vi "Controller LNLS Control BPM Communication Loop.vi"(7 "Sync Objects":T1, 8 "error in (no error)":errorcluster, 11 "FOFB Configuration":T4={"FOFB Parameters"={"Network"={"FOFB Controller IP"="", "LNLS Control Network IP"="", "LNLS Control Network Power Supplies TCP Port"=0, "LNLS Control Network FOFB Configuration TCP Port"=0, "LNLS Control Network BPMs TCP Port"=0, "Data Server TCP Port"=0, "Monitoring Data TCP Port"=0, "Configuration GUI TCP Port"=0, "Storage Data TCP Port"=0, "Fast Command TCP Port"=0, "TCP Listening Timeout"=0, "Request Setpoints Rate"=0}, "Fast Acquisition"={"Acquisition Period"=0, "Data Buffer Size"=0, "Monitoring Period"=0}, "Response Matrix Measurement"={"Step Amplitude"=0.0, "Time Between Steps"=0, "Step Duration"=0, "Number of Averages"=0}, "Correction Algorithm"={"Correction Period"=0, "Reference Orbit Path"=path "", "Response Matrix Path"=path "", "Correction Matrix Path"=path "", "PID Horizontal Gain"=0.0, "PID Vertical Gain"=0.0, "PID Horizontal Integral Time"=0.0, "PID Vertical Integral Time"=0.0, "PID Horizontal Derivative Time"=0.0, "PID Vertical Derivative Time"=0.0, "Beam Current FOFB Threshold"=0.0, "Decouple H-V"=FALSE, "Use Additional BPM LPF"=FALSE, "BPM LPF Cutoff"=0.0}, "Acquisition Network"=[], "Actuation Network"=[]}, "Number of Acquisition Chassis"=0, "Number of Actuation Chassis"=0, "Number of BPM Readings"=0, "BPM Reading Names"=[], "Selected BPM Readings"=[0, 1, 2, 3, 4, 5, 6, 7, 8, 9, 10, 11, 12, 13, 14, 15, 16, 17, 18, 19, 20, 21, 22, 23, 24, 25, 26, 27, 28, 29, 30, 31, 32, 33, 34, 35, 36, 37, 38, 39, 40, 41, 42, 43, 44, 45, 46, 47, 48, 49], "Number of Correctors"=0, "Corrector Names"=[], "Selected Correctors"=[0, 1, 2, 3, 4, 5, 6, 7, 8, 9, 10, 11, 12, 13, 14, 15, 16, 17, 18, 19, 20, 21, 22, 23, 24, 25, 26, 27, 28, 29, 30, 31, 32, 33, 34, 35, 36, 37, 38, 39, 40, 41, 42, 43, 44, 45, 46, 47, 48, 49], "Reference Orbit"=[], "Response Matrix"=[], "Correction Matrix"=[], "Acquisition Chassis Names"=[], "Actuation Chassis Names"=[], "Acquisition Variables"=[], "Actuation Variables"=[], "PS Matrix Mapping"=[], "Inverse PS Matrix Mapping"=[], "BPM Matrix Mapping"=[], "Inverse BPM Matrix Mapping"=[], "Response Matrix Beam Energy (MeV)"=0.0, "PID Parameters"=[], "BPM Planes"=[], "Corrector Planes"=[], "RMM Step Factor"=[]}) -> (0 "error out":errorcluster)   [LabVIEW 2011, in "Controller Global Variables.lvlib"]
uses:
  Controller Global Variables.lvlib
  Types Definitions/Type FOFB Configuration.ctl
  Types Definitions/Type FOFB Parameters.ctl
  Types Definitions/Type Network Configuration.ctl
  Types Definitions/Type FA Configuration.ctl
  Types Definitions/Type Response Matrix Measurement Configuration.ctl
  Types Definitions/Type Correction Algorithm Configuration.ctl
  Types Definitions/Type Acquisition Network Configuration.ctl
  Types Definitions/Type Actuation Network Configuration.ctl
  Types Definitions/Type PID Parameters.ctl
  Types Definitions/Type Synchronization Objects.ctl
  Types Definitions/Type Blocking Synchronization Objects.ctl
  Types Definitions/Type Monitoring Data.ctl
  Types Definitions/Type Operation Mode State.ctl
  Types Definitions/Type Diagnostics Data.ctl
  Types Definitions/Type CPU Loads Array.ctl
  Types Definitions/Type CPU Loads.ctl
  Types Definitions/Type Non-blocking Synchronization Objects.ctl
  Types Definitions/Type FOFB Variables.ctl
  Types Definitions/Type Actuation State.ctl
  Types Definitions/Type TCP State.ctl
  <vilib>/Platform/TimedLoop/XDataNode/timing_clust.ctl
  <vilib>/Platform/TimedLoop/XDataNode/nitl_modes.ctl
  <vilib>/Platform/TimedLoop/XDataNode/wakeup.ctl
  Controller Global Variables/Monitoring Data.vi
  <vilib>/Platform/TimedLoop/XDataNode/XDataNode.xnode
  Type Definitions.lvlib
  LNLS Control VIs.lvlib
  Misc VIs.lvlib
  <vilib>/Platform/TimedLoop/XDataNode/XDNodeRunTimeDep.lvlib
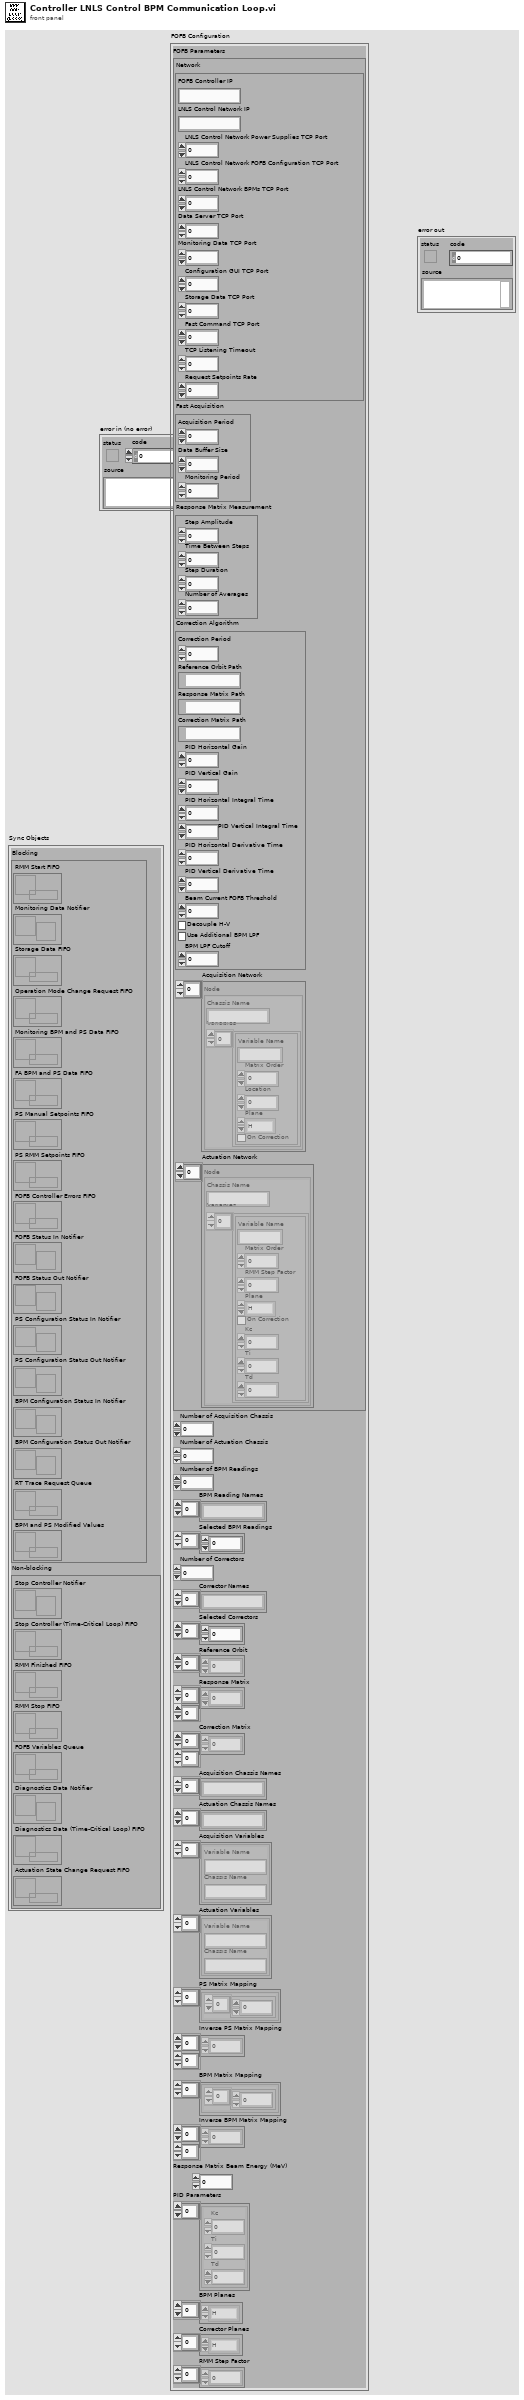
[diagram p1: front panel]
types:
  T1 = typedef "Type Definitions.lvlib/Type Synchronization Objects.ctl" = cluster{"Blocking":T2, "Non-blocking":T3}
  T2 = typedef "Type Definitions.lvlib/Type Blocking Synchronization Objects.ctl" = cluster{"RMM Start FIFO":refnum<k33>, "Monitoring Data Notifier":refnum<notifier>, "Storage Data FIFO":refnum<queue>, "Operation Mode Change Request FIFO":refnum<k33>, "Monitoring BPM and PS Data FIFO":refnum<k33>, "FA BPM and PS Data FIFO":refnum<k33>, "PS Manual Setpoints FIFO":refnum<k33>, "PS RMM Setpoints FIFO":refnum<k33>, "FOFB Controller Errors FIFO ":refnum<k33>, "FOFB Status In Notifier":refnum<notifier>, "FOFB Status Out Notifier":refnum<notifier>, "PS Configuration Status In Notifier":refnum<notifier>, "PS Configuration Status Out Notifier":refnum<notifier>, "BPM Configuration Status In Notifier":refnum<notifier>, "BPM Configuration Status Out Notifier":refnum<notifier>, "RT Trace Request Queue":refnum<queue>, "BPM and PS Modified Values":refnum<k33>}
  T3 = typedef "Type Definitions.lvlib/Type Non-blocking Synchronization Objects.ctl" = cluster{"Stop Controller Notifier":refnum<notifier>, "Stop Controller (Time-Critical Loop) FIFO":refnum<k33>, "RMM Finished FIFO":refnum<k33>, "RMM Stop FIFO":refnum<k33>, "FOFB Variables Queue":refnum<queue>, "Diagnostics Data Notifier":refnum<notifier>, "Diagnostics Data (Time-Critical Loop) FIFO":refnum<k33>, "Actuation State Change Request FIFO":refnum<k33>}
  T4 = typedef "Type Definitions.lvlib/Type FOFB Configuration.ctl" = cluster{"FOFB Parameters":T5, "Number of Acquisition Chassis":i32, "Number of Actuation Chassis":i32, "Number of BPM Readings":i32, "BPM Reading Names":string[], "Selected BPM Readings":u32[], "Number of Correctors":i32, "Corrector Names":string[], "Selected Correctors":u32[], "Reference Orbit":dbl[], "Response Matrix":dbl[][], "Correction Matrix":dbl[][], "Acquisition Chassis Names":string[], "Actuation Chassis Names":string[], "Acquisition Variables":cluster{"Variable Name":string, "Chassis Name":string}[], "Actuation Variables":cluster{"Variable Name":string, "Chassis Name":string}[], "PS Matrix Mapping":cluster{u32[]}[], "Inverse PS Matrix Mapping":u32[][], "BPM Matrix Mapping":cluster{u32[]}[], "Inverse BPM Matrix Mapping":u32[][], "Response Matrix Beam Energy (MeV)":dbl, "PID Parameters":T12[], "BPM Planes":enum8{"H", "V"}[], "Corrector Planes":enum8{"H", "V"}[], "RMM Step Factor":dbl[]}
  T5 = typedef "Type Definitions.lvlib/Type FOFB Parameters.ctl" = cluster{"Network":T6, "Fast Acquisition":T7, "Response Matrix Measurement":T8, "Correction Algorithm":T9, "Acquisition Network":T10, "Actuation Network":T11}
  T6 = typedef "Type Definitions.lvlib/Type Network Configuration.ctl" = cluster{"FOFB Controller IP":string, "LNLS Control Network IP":string, "LNLS Control Network Power Supplies TCP Port":u16, "LNLS Control Network FOFB Configuration TCP Port":u16, "LNLS Control Network BPMs TCP Port":u16, "Data Server TCP Port":u16, "Monitoring Data TCP Port":u16, "Configuration GUI TCP Port":u16, "Storage Data TCP Port":u16, "Fast Command TCP Port":u16, "TCP Listening Timeout":i32, "Request Setpoints Rate":u16}
  T7 = typedef "Type Definitions.lvlib/Type FA Configuration.ctl" = cluster{"Acquisition Period":u32, "Data Buffer Size":u32, "Monitoring Period":u32}
  T8 = typedef "Type Definitions.lvlib/Type Response Matrix Measurement Configuration.ctl" = cluster{"Step Amplitude":dbl, "Time Between Steps":u32, "Step Duration":u32, "Number of Averages":u32}
  T9 = typedef "Type Definitions.lvlib/Type Correction Algorithm Configuration.ctl" = cluster{"Correction Period":u32, "Reference Orbit Path":path, "Response Matrix Path":path, "Correction Matrix Path":path, "PID Horizontal Gain":dbl, "PID Vertical Gain":dbl, "PID Horizontal Integral Time":dbl, "PID Vertical Integral Time":dbl, "PID Horizontal Derivative Time":dbl, "PID Vertical Derivative Time":dbl, "Beam Current FOFB Threshold":dbl, "Decouple H-V":bool, "Use Additional BPM LPF":bool, "BPM LPF Cutoff":dbl}
  T10 = typedef "Type Definitions.lvlib/Type Acquisition Network Configuration.ctl" = cluster{"Chassis Name":string, "Variables":cluster{"Variable Name":string, "Matrix Order":u32, "Location":dbl, "Plane":enum8{"H", "V"}, "On Correction":bool}[]}[]
  T11 = typedef "Type Definitions.lvlib/Type Actuation Network Configuration.ctl" = cluster{"Chassis Name":string, "Variables":cluster{"Variable Name":string, "Matrix Order":u32, "RMM Step Factor":dbl, "Plane":enum8{"H", "V"}, "On Correction":bool, "Kc":dbl, "Ti":dbl, "Td":dbl}[]}[]
  T12 = typedef "Type Definitions.lvlib/Type PID Parameters.ctl" = cluster{"Kc":fxp<+/-,16,8>, "Ti":fxp<+/-,16,8>, "Td":fxp<+/-,16,8>}
  T13 = typedef "Type Definitions.lvlib/Type TCP State.ctl" = enum16{"Idle", "Wait Connection", "Read Data", "Process Data", "Write Data", "Close Connection"}
  T14 = typedef "XDNodeRunTimeDep.lvlib/timing_clust.ctl" = cluster{"Expected End [f-1]":u64, "Actual End [f-1]":u64, "Finished Late? [f-1]":bool, "Expected End [i-1]":u64, "Actual End [i-1]":u64, "Finished Late? [i-1]":bool, "Expected Start [i]":u64, "Actual Start [i]":u64, "Expected Start [f]":u64, "Actual Start [f]":u64, "Source Name":string, "Structure Name":string, "Period":i64, "Deadline":i64, "Offset":i64, "Start":i64, "Priority":i32, "Timeout":i32, "Mode":T15, "Wakeup Reason":T16, "Error":errorcluster, "Source Type":string, "Secondary Source Type":string, "Global End Time":u64, "Global Start Time":u64, "Frame Duration":u64, "Iteration Duration":u64, "Assigned CPU":i32, "I/O Scan Engine Mode":u32}
  T15 = typedef "XDNodeRunTimeDep.lvlib/nitl_modes.ctl" = enum32{"No Change", "Process missed periods, maintain original phase", "Discard missed periods, maintain original phase", "Process missed periods, ignore original phase", "Discard missed periods, ignore original phase"}
  T16 = typedef "XDNodeRunTimeDep.lvlib/wakeup.ctl" = enum32{"Normal", "Aborted", "Asynchronous wakeup", "Timing source error", "Timed loop error", "Timeout"}
  T17 = typedef "Type Definitions.lvlib/Type Monitoring Data.ctl" = cluster{"Timestamp":timestamp, "BPM Readings":dbl[], "PS Readings":dbl[], "PS FOFB Setpoints":dbl[], "PS Status per Rack":u8[], "PS ON-OFF per Rack":u8[], "Operation Mode":T18, "Diagnostics Data":T19, "Controller Status Table":i32[]}
  T18 = typedef "Type Definitions.lvlib/Type Operation Mode State.ctl" = enum8{"Idle Mode", "Manual Mode", "FOFB Mode", "RMM Mode"}
  T19 = typedef "Type Definitions.lvlib/Type Diagnostics Data.ctl" = cluster{"Time-Critical Loop Missed Iterations":u32, "Time-Critical Loop Execution Time (usec)":u32, "Available Memory (bytes)":u32, "CPU Loads Array":T20}
  T20 = typedef "Type Definitions.lvlib/Type CPU Loads Array.ctl" = T21[]
  T21 = typedef "Type Definitions.lvlib/Type CPU Loads.ctl" = cluster{"Total (%)":dbl, "Time Critical (%)":dbl, "Timed Structures (%)":dbl, "High (%)":dbl, "Above Normal (%)":dbl, "Normal (%)":dbl, "Background (%)":dbl, "Idle (%)":dbl, "ISR (%)":dbl}
  T22 = typedef "Type Definitions.lvlib/Type BPM Pre Encode.ctl" = cluster{"analog value":dbl, "status":u8}
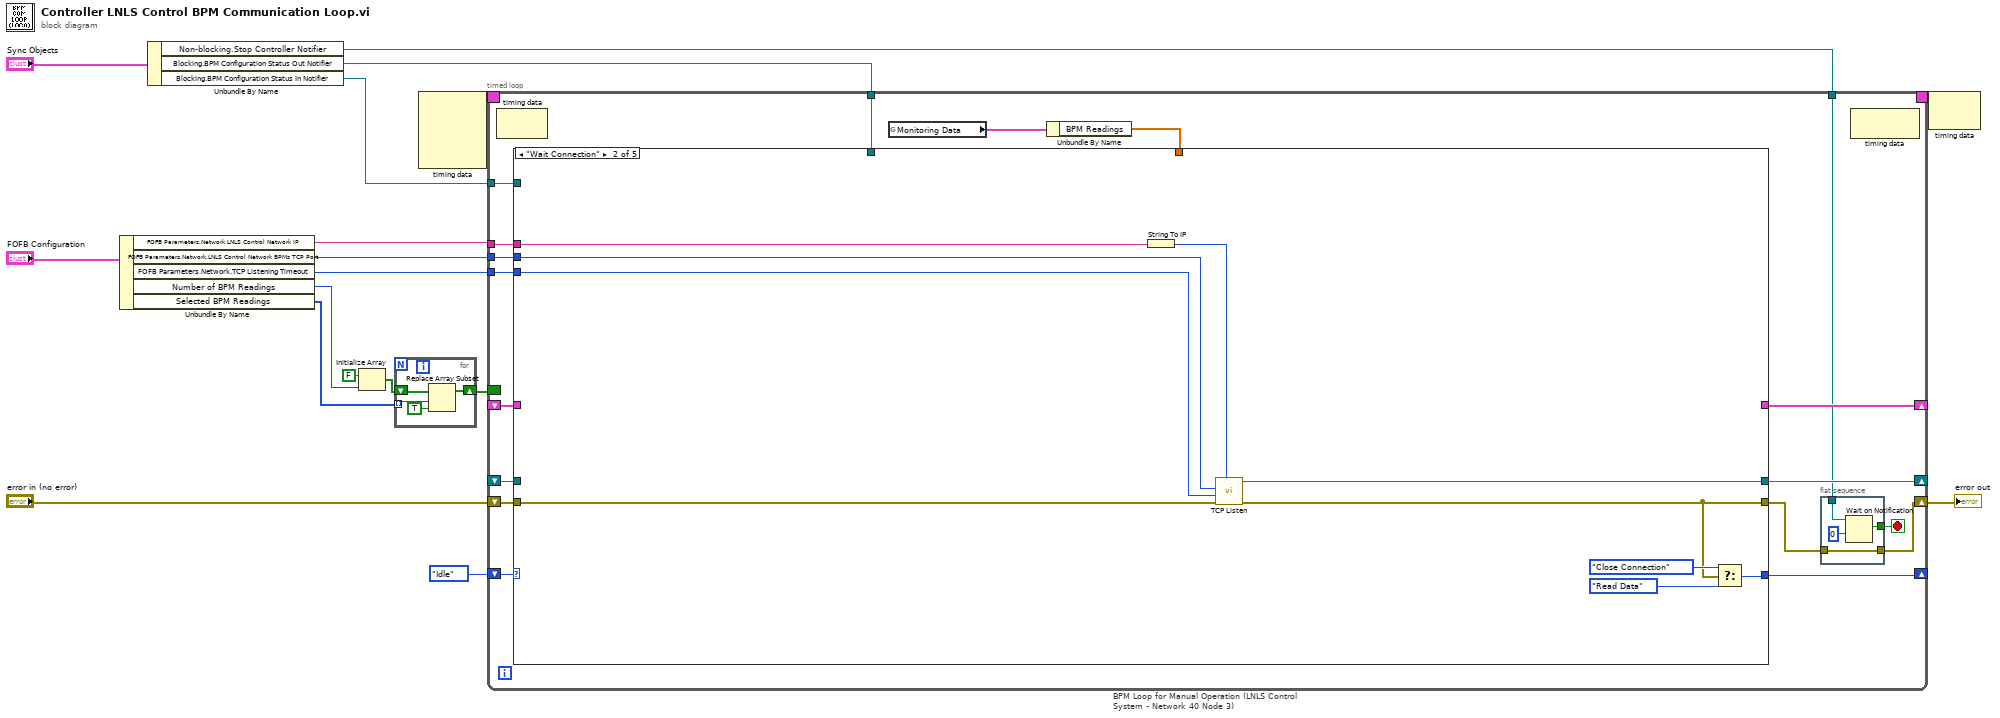
[diagram p0: block diagram]
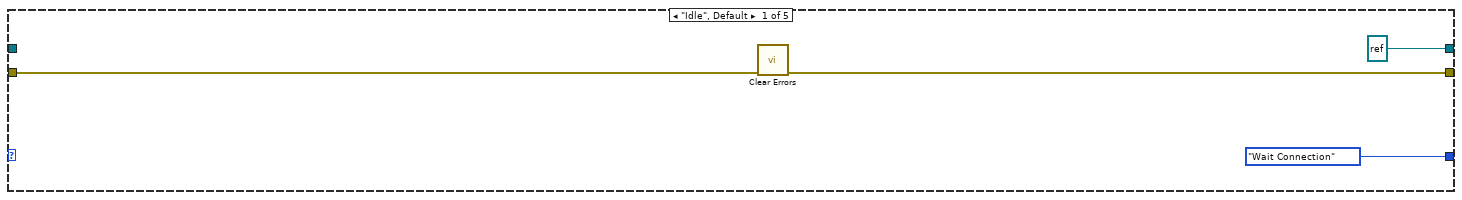
[diagram p2: hidden frame]
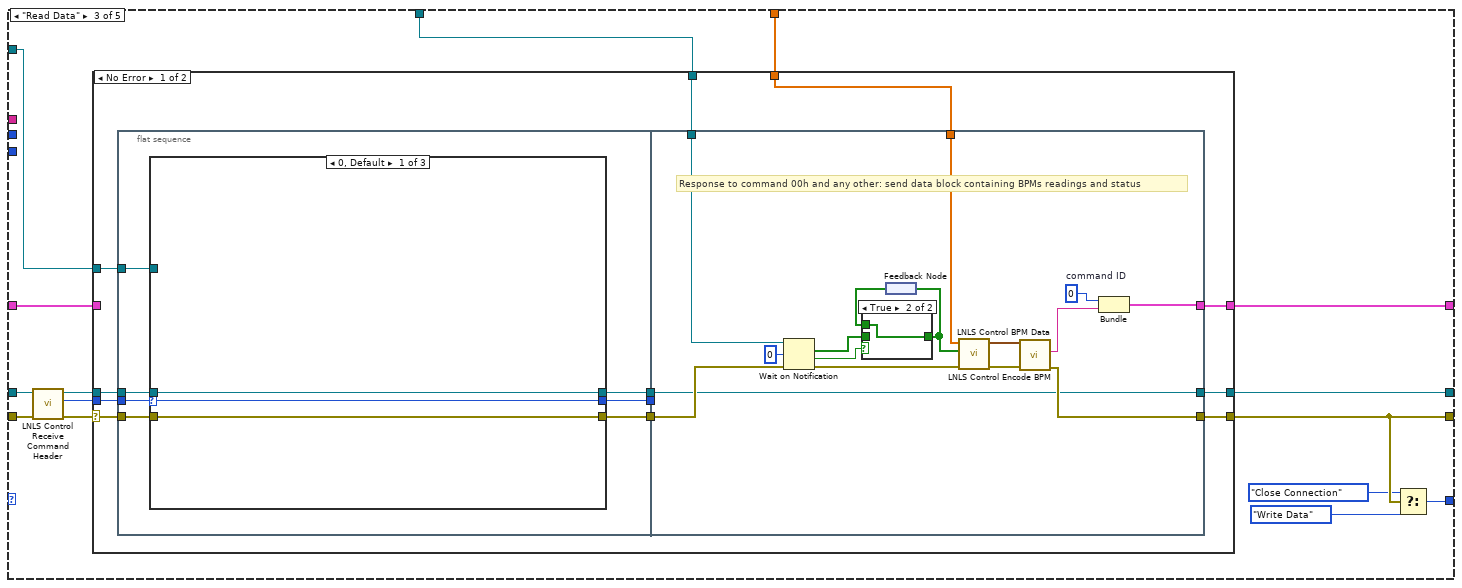
[diagram p3: hidden frame]
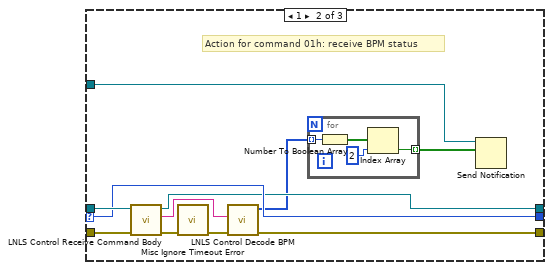
[diagram p4: hidden frame]
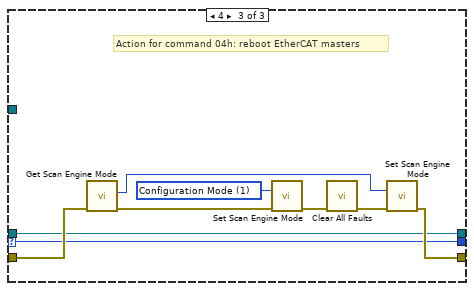
[diagram p5: hidden frame]
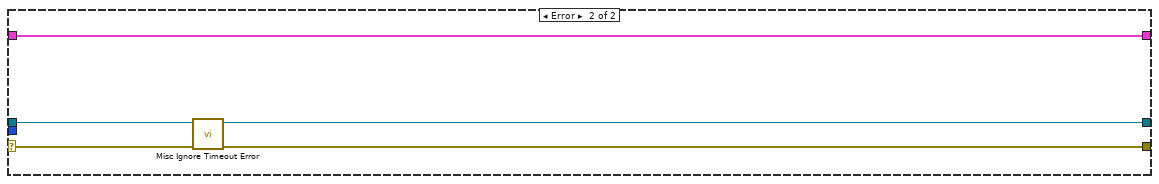
[diagram p7: hidden frame]
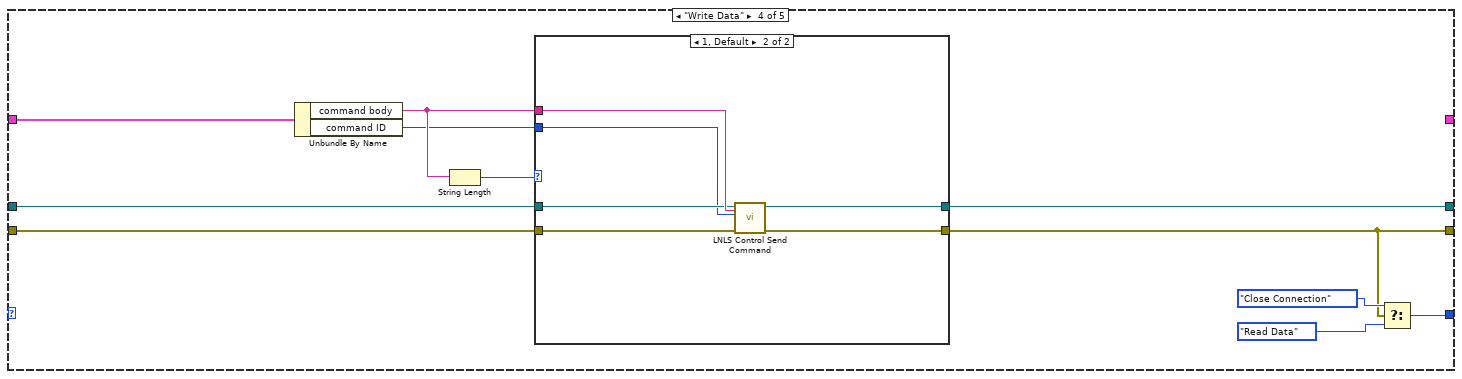
[diagram p8: hidden frame]
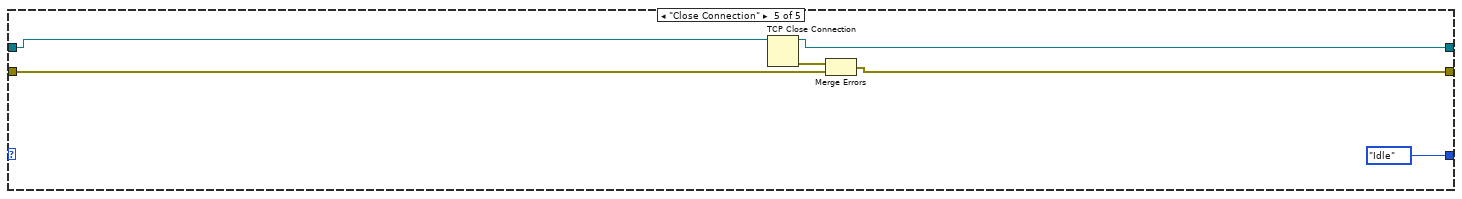
[diagram p10: hidden frame]
diagram:
  n1 = Unbundle By Name("FOFB Configuration") -> ("FOFB Parameters.Network.LNLS Control Network IP"=w11:string, "FOFB Parameters.Network.LNLS Control Network BPMs TCP Port"=w10:u16, "FOFB Parameters.Network.TCP Listening Timeout"=w9:i32, "Number of BPM Readings"=w3:i32, "Selected BPM Readings"=w2:u32[])
  n2 = Unbundle By Name("Sync Objects") -> ("Non-blocking.Stop Controller Notifier"=w7:refnum<notifier>, "Blocking.BPM Configuration Status Out Notifier"=w6:refnum<notifier>, "Blocking.BPM Configuration Status In Notifier"=w8:refnum<notifier>)
  n3 = Initialize Array(FALSE, w3) -> (w4:bool[])
  n4 = for {
    tunnel: w2 -> [w22] mode=indexing
    shift-right: [w19] -> w1
    shift-left: w4 -> [w21]
    n5 = Replace Array Subset(array=w21, new element=TRUE ("new element/subarray"), index=w22) -> (w19:bool[])
  }
  n6 = node-c288() -> (w18:T14)  [unwired: 4 in]
  n7 = timed-loop "BPM Loop for Manual Operation (LNLS Control System - Network 40 Node 3)" {
    shift-right: [w38] -> _
    shift-left: Type_TCP_State."Idle" ("f") -> [w40]
    shift-right: [w39] -> _
    shift-left: _ -> [w37]
    shift-right: [w28] -> w14
    shift-left: "error in (no error)" -> [w33]
    shift-right: [w35] -> _
    shift-left: _ -> [w34]
    tunnel: w10 -> [w36]
    tunnel: w11 -> [w32]
    tunnel: w7 -> [w30]
    tunnel: w9 -> [w31]
    timing: w18 -> [_]
    timing-out: [_] -> w17
    tunnel: w8 -> [w25]
    tunnel: w6 -> [w24]
    border: w1 -> [_]
    stop <- w29 stop-if-true
    n8 = node-c288() -> ()  [unwired: 1 in, 1 out]
    n9 = global read "Monitoring Data.vi" "Monitoring Data"() -> (w27:T17)
    n10 = Unbundle By Name(w27) -> ("BPM Readings"=w26:dbl[])
    n11 = case shown="\"Wait Connection\"" w40 {
      tunnel: [refnum<k5> refnum ("connection ID") w57 w75 w147 w167] -> w39
      tunnel: [w48 w52 w73 w146 w163] -> w23
      tunnel: [Type_TCP_State."Wait Connection" w60 w74 w152 Type_TCP_State."Idle"] -> w38
      tunnel: w37 -> [_ _ w71 w149 w168]
      tunnel: w33 -> [w47 w53 w72 w148 w165]
      tunnel: w36 -> [_ w56 _ _ _]
      tunnel: [_ _ w68 _ _] -> w35
      tunnel: w34 -> [_ _ w66 w151 _]
      tunnel: w32 -> [_ w54 _ _ _]
      tunnel: w31 -> [_ w51 _ _ _]
      tunnel: w26 -> [_ _ w63 _ _]
      tunnel: w25 -> [_ _ w62 _ _]
      tunnel: w24 -> [_ _ w61 _ _]
      frame "Idle", Default {
        n12 = call <vilib>:"Clear Errors.vi"("error in (no error)"=w47) -> ("error out"=w48:errorcluster)  [unwired: 6 in]
      }
      frame "Wait Connection" {
        n13 = String To IP(1:w54) -> (0:w55:u32)
        n14 = call <vilib>:"TCP Listen.vi"("net address"=w55, "error in (no error)"=w53, "timeout ms (wait forever: -1)"=w51, "port"=w56) -> ("error out"=w52:errorcluster, "connection ID"=w57:refnum<k5>)  [unwired: 3 in, 3 out]
        n15 = Select(t=Type_TCP_State."Close Connection", s=w52, f=Type_TCP_State."Read Data") -> (s? t:f=w60:T13)
      }
      frame "Read Data" {
        n16 = call "LNLS Control Receive Command Header.vi"("error in (no error)"=w72, "connection ID"=w71) -> ("error out"=w67:errorcluster, "command ID"=w64:u8, "connection ID out"=w70:refnum<k5>)  [unwired: 7 in]
        n17 = case shown="No Error" w67 {
          selector: w67 -> [w82 w140]
          tunnel: [w87 w143] -> w75
          tunnel: [w86 w141] -> w73
          tunnel: w70 -> [w85 w143]
          tunnel: w64 -> [w84 _]
          tunnel: [w83 w142] -> w68
          tunnel: w66 -> [_ w142]
          tunnel: w63 -> [w78 _]
          tunnel: w62 -> [w77 _]
          tunnel: w61 -> [w76 _]
          frame No Error {
            n18 = flat-sequence {
              tunnel: [w94] -> w81
              tunnel: [w93] -> w80
              tunnel: w85 -> [w92]
              tunnel: w84 -> [w91]
              tunnel: w82 -> [w90]
              tunnel: [w89] -> w79
              tunnel: w77 -> [w88]
              tunnel: [w135] -> w87
              tunnel: w81 -> [w135]
              tunnel: [w137] -> w86
              tunnel: w80 -> [w136]
              tunnel: [w134] -> w83
              tunnel: w79 -> [_]
              tunnel: w78 -> [w128]
              tunnel: w76 -> [w133]
              frame #0 {
                n19 = case shown="0, Default" w91 {
                  selector: w91 -> [w95 w106 w114]
                  tunnel: w90 -> [w97 w107 w121]
                  tunnel: [w97 w98 w120] -> w93
                  tunnel: [w96 w105 w113] -> w94
                  tunnel: w92 -> [w96 w108 w113]
                  tunnel: [w95 w106 w114] -> w89
                  tunnel: w88 -> [_ w99 _]
                  frame 0, Default {
                  }
                  frame 1 {
                    # "Action for command 01h: receive BPM status"
                    n20 = call "LNLS Control Receive Command Body.vi"("error in (no error)"=w107, "connection ID"=w108) -> ("error out"=w104:errorcluster, "command body"=w103:string, "connection ID out"=w105:refnum<k5>)  [unwired: 6 in, 1 out]
                    n21 = call "Misc Ignore Timeout Error.vi"("error in (no error)"=w104) -> ("error out"=w102:errorcluster)  [unwired: 9 in, 1 out]
                    n22 = call "LNLS Control Decode BPM.vi"("error in (no error)"=w102, "command body"=w103) -> ("error out"=w98:errorcluster, "BPM Control"=w100:u8[])  [unwired: 6 in]
                    n23 = for {
                      tunnel: w100 -> [w112] mode=indexing
                      tunnel: [w109] -> w101 mode=indexing
                      n24 = Number To Boolean Array(number=w112) -> (Boolean array=w111:bool[])
                      n25 = Index Array(array=w111, index=2) -> (element=w109:bool)
                    }
                    n26 = Send Notification(notification=w101, notifier=w99) -> ()  [unwired: 1 in, 2 out]
                  }
                  frame 4 {
                    w119 = 1 items=["Configuration Mode"=1, "Active Mode"=2] ("mode (Active Mode)")
                    # "Action for command 04h: reboot EtherCAT masters"
                    n27 = call <vilib>:"Get Scan Engine Mode.vi"("error in (no error)"=w121) -> ("error out"=w118:errorcluster, "mode"=w115:i32)  [unwired: 9 in]
                    n28 = call <vilib>:"Set Scan Engine Mode.vi"("mode (Active Mode)"=w119, "error in (no error)"=w118) -> ("error out"=w117:errorcluster)  [unwired: 13 in]
                    n29 = call <vilib>:"Clear All Faults.vi"("error in (no error)"=w117) -> ("error out"=w116:errorcluster)  [unwired: 1 in, 9 out]
                    n30 = call <vilib>:"Set Scan Engine Mode.vi"("mode (Active Mode)"=w115, "error in (no error)"=w116) -> ("error out"=w120:errorcluster)  [unwired: 13 in]
                  }
                }
              }
              frame #1 {
                w132 = u8 0  # command ID
                # "Response to command 00h and any other: send data block containing BPMs readings and status"
                n31 = Wait on Notification(notifier=w133, timeout in ms (-1)=0, error in (no error)=w136) -> (notification=w125:bool[], timed out?=w126:bool, error out=w129:errorcluster)  [unwired: 1 in, 1 out]
                n32 = feedback #1() -> (w123:bool[])
                n33 = case shown="True" w126 {
                  tunnel: w125 -> [w138 _]
                  tunnel: [w138 w139] -> w122
                  tunnel: w123 -> [_ w139]
                  frame False {
                  }
                  frame True {
                  }
                }
                n34 = feedback-in #1(w122) -> ()
                n35 = call "LNLS Control BPM Data.vi"("error in (no error)"=w129, "BPM Status (On correction?)"=w122, "BPM Readings"=w128) -> ("error out"=w131:errorcluster, "BPM Readings Data"=w127:T22[])  [unwired: 7 in]
                n36 = call "LNLS Control Encode BPM.vi"("error in (no error)"=w131, "BPM Data"=w127) -> ("error out"=w137:errorcluster, "command body"=w130:string)  [unwired: 8 in]
                n37 = Bundle("command ID"=w132, "command body"=w130) -> (w134:cluster{"command ID":u8, "command body":string})  [unwired: 1 in]
              }
            }
          }
          frame Error {
            n38 = call "Misc Ignore Timeout Error.vi"("error in (no error)"=w140) -> ("error out"=w141:errorcluster)  [unwired: 9 in, 1 out]
          }
        }
        n39 = Select(t=Type_TCP_State."Close Connection", s=w73, f=Type_TCP_State."Write Data") -> (s? t:f=w74:T13)
      }
      frame "Write Data" {
        n40 = Unbundle By Name(w151) -> ("command body"=w150:string, "command ID"=w145:u8)
        n41 = String Length(string=w150) -> (length=w144:i32)
        n42 = case shown="1, Default" w144 {
          tunnel: w150 -> [_ w162]
          tunnel: w149 -> [w156 w161]
          tunnel: w148 -> [w155 w160]
          tunnel: [w156 w159] -> w147
          tunnel: [w155 w158] -> w146
          tunnel: w145 -> [_ w157]
          frame 0 {
          }
          frame 1, Default {
            n43 = call "LNLS Control Send Command.vi"("command body"=w162, "error in (no error)"=w160, "command ID"=w157, "connection ID"=w161) -> ("error out"=w158:errorcluster, "connection ID out"=w159:refnum<k5>)  [unwired: 6 in]
          }
        }
        n44 = Select(t=Type_TCP_State."Close Connection", s=w146, f=Type_TCP_State."Read Data") -> (s? t:f=w152:T13)
      }
      frame "Close Connection" {
        n45 = TCP Close Connection(connection ID=w168) -> (connection ID out=w167:refnum<k5>, error out=w164:errorcluster)  [unwired: 2 in]
        n46 = Merge Errors(w164, w165) -> (w163:errorcluster)
      }
    }
    n47 = flat-sequence {
      tunnel: w30 -> [w45]
      tunnel: [w43] -> w28
      tunnel: [w44] -> w29
      tunnel: w23 -> [w43]
      frame #0 {
        n48 = Wait on Notification(notifier=w45, timeout in ms (-1)=0) -> (notification=w44:bool)  [unwired: 2 in, 3 out]
      }
    }
    n49 = node-c288() -> ()  [unwired: 1 in, 1 out]
  }
  "error out" <- w14
  n50 = node-c288(w17) -> ()  [unwired: 1 out]
